vi "onDestroyDebugTerminal.vi"(8 "error in (no error)":errorcluster, 11 "DebuggingTerminal in":refnum<class "DebuggingTerminal.lvclass">) -> (0 "error out":errorcluster, 3 "DebuggingTerminal out":refnum<class "DebuggingTerminal.lvclass">)   [LabVIEW 2013, in "MQTT Base.lvlib" / "DebuggingTerminal.lvclass"]
uses:
  DebuggingTerminal.lvclass
  DebuggingTerminal.lvclass/DebuggingTerminal.ctl
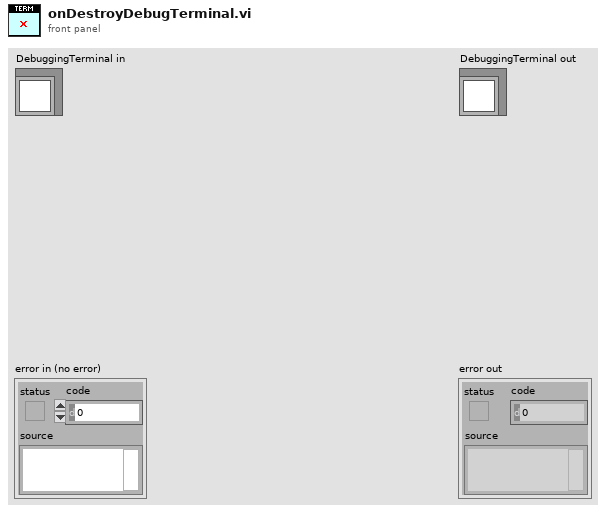
[diagram p1: front panel]
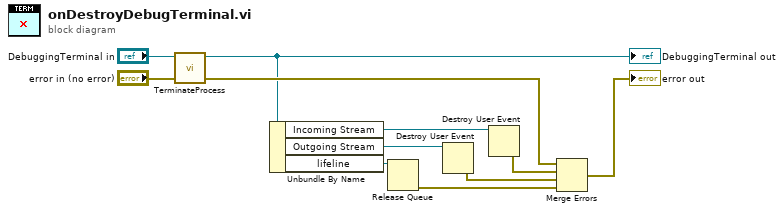
[diagram p0: block diagram]
diagram:
  n1 = call "TerminateProcess.vi"("DebuggingTerminal in"="DebuggingTerminal in") -> ("DebuggingTerminal out"=w1:refnum<class "DebuggingTerminal.lvclass">)  [unwired: 10 in]
  "DebuggingTerminal out" <- w1
  n2 = Unbundle By Name(w1) -> ("Incoming Stream"=w10:refnum<user-event>, "Outgoing Stream"=w9:refnum<user-event>, "lifeline"=w3:refnum<queue>)
  n3 = Release Queue(queue=w3) -> (error out=w6:errorcluster)  [unwired: 2 in, 2 out]
  n4 = Destroy User Event(user event=w9) -> (error out=w5:errorcluster)  [unwired: 1 in]
  n5 = Destroy User Event(user event=w10) -> (error out=w4:errorcluster)  [unwired: 1 in]
  n6 = Merge Errors("error in (no error)", w4, w5, w6) -> (→"error out":errorcluster)
